vi "Reset.vi"(8 "error in (no error)":errorcluster, 11 "TileTimer in":refnum<class "TileTimer.lvclass">) -> (0 "error out":errorcluster, 3 "TileTimer out":refnum<class "TileTimer.lvclass">)   [LabVIEW 2019, in "RT_Game.lvlib" / "TileTimer.lvclass"]
uses:
  TileTimer.lvclass
  TileTimer.lvclass/TileTimer.ctl
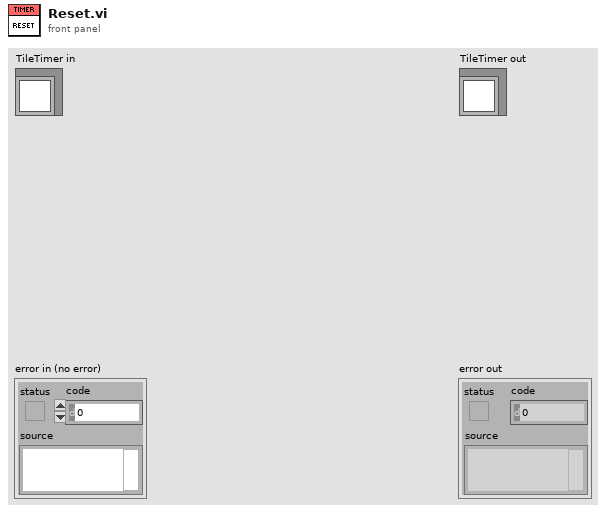
[diagram p1: front panel]
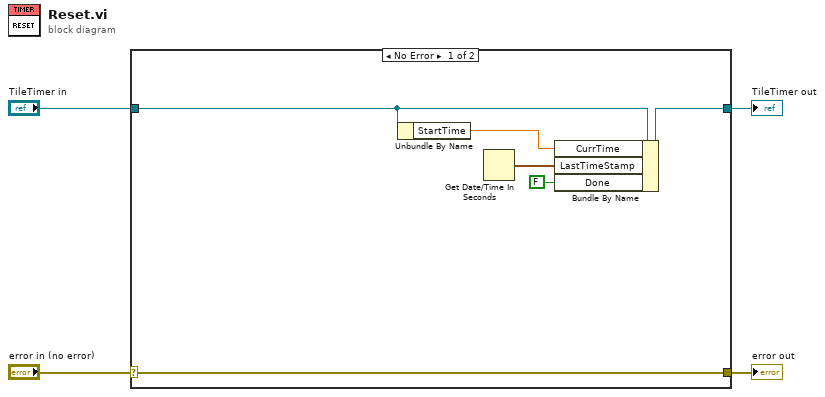
[diagram p0: block diagram]
diagram:
  n1 = case shown="No Error" "error in (no error)" {
    selector: "error in (no error)" -> [w10 w12]
    tunnel: [w10 w12] -> w3
    tunnel: [w9 w11] -> w1
    tunnel: "TileTimer in" -> [w7 w11]
    frame No Error {
      n2 = Unbundle By Name(w7) -> ("StartTime"=w6:dbl)
      n3 = Get Date/Time In Seconds() -> (seconds since 1Jan1904=w8:timestamp)
      n4 = Bundle By Name(cluster=w7, "CurrTime"=w6, "LastTimeStamp"=w8, "Done"=FALSE) -> (w9:refnum<class "TileTimer.lvclass">)
    }
    frame Error {
    }
  }
  "error out" <- w3
  "TileTimer out" <- w1
